vi "Enumerate COMM Address.vi"(8 "error in (no error)":errorcluster, 11 "Hardware in":refnum<class "Hardware.lvclass">) -> (0 "error out":errorcluster, 2 "Array of COMM Addresses":string[](array[string]), 3 "Hardware out":refnum<class "Hardware.lvclass">)   [LabVIEW 2016, in "Hardware.lvlib" / "Hardware.lvclass"]
uses:
  <userlib>/Common Components/Hardware/Abstract Hardware/Hardware.lvclass
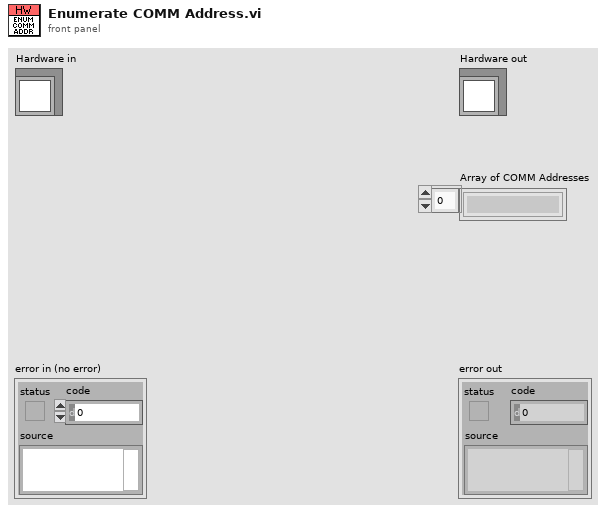
[diagram p1: front panel]
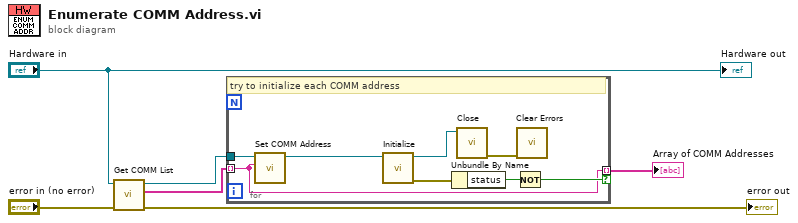
[diagram p0: block diagram]
diagram:
  n1 = call-dynamic "Get COMM List.vi"("error in (no error)"="error in (no error)", "Hardware in"="Hardware in") -> ("error out"=→"error out":errorcluster, "COMM List"=w2:string[], "Hardware out"=w3:refnum<class "Hardware.lvclass">)  [unwired: 7 in]
  n2 = for {
    tunnel: w3 -> [w9]
    tunnel: w2 -> [w7] mode=indexing
    tunnel: [w7] -> w1 mode=indexing if=w12
    # "try to initialize each COMM address"
    n3 = call <userlib>:"Set COMM Address.vi"("COMM Address"=w7, "Hardware in"=w9) -> ("Hardware out"=w8:refnum<class "Hardware.lvclass">)  [unwired: 8 in, 1 out]
    n4 = call-dynamic "Initialize.vi"("Hardware in"=w8) -> ("error out"=w14:errorcluster, "Hardware out"=w11:refnum<class "Hardware.lvclass">)  [unwired: 9 in]
    n5 = Unbundle By Name(w14) -> ("status"=w13:bool)
    n6 = call-dynamic "Close.vi"("Hardware in"=w11) -> ("error out"=w10:errorcluster)  [unwired: 9 in, 1 out]
    n7 = Not(x=w13) -> (.not. x?=w12:bool)
    n8 = call <vilib>:"Clear Errors.vi"("error in (no error)"=w10) -> ()  [unwired: 5 in, 2 out]
  }
  "Array of COMM Addresses" <- w1
  "Hardware out" <- "Hardware in"
